vi "Exit if Runtime.vi"(3 "Top Level VI reference":refnum<vi>) -> ()   [LabVIEW 2026]
panel:
  in  "error in (no error)":errorcluster
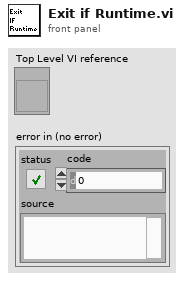
[diagram p1: front panel]
types:
  T1 = enum32{"invalid app kind", "Development System", "Run Time System", "Student Edition", "Embedded LabVIEW", "Evaluation", "Custom"}
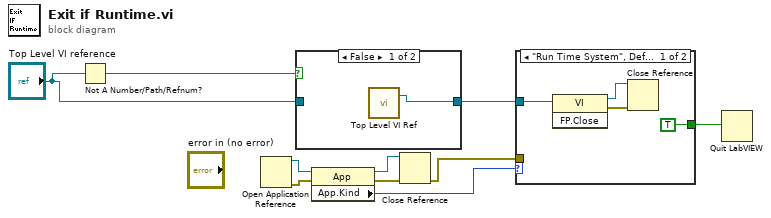
[diagram p0: block diagram]
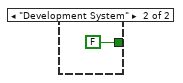
[diagram p2: hidden frame]
diagram:
  n1 = Not A Number/Path/Refnum?(number/path/refnum="Top Level VI reference") -> (NaN/Path/Refnum?=w10:bool)
  n2 = Open Application Reference() -> (0:w4:errorcluster, 3:w3:refnum<vi>)  [unwired: 4 in]
  n3 = case shown="False" w10 {
    tunnel: "Top Level VI reference" -> [_ w12]
    tunnel: [w11 w12] -> w2
    frame False {
      n4 = call "Top Level VI Ref.vi"() -> ("Top Level VI reference"=w11:refnum<vi>)  [unwired: 3 in]
    }
    frame True {
    }
  }
  n5 = property class="App"(reference=w3, error in=w4) -> (reference out=w5:refnum<vi>, error out=w8:errorcluster, "App.Kind"=w7:T1)
  n6 = Close Reference(reference=w5, error in (no error)=w8) -> (error out=w6:errorcluster)
  n7 = case shown="\"Run Time System\", Default" w7 {
    tunnel: w6 -> [_ _]
    tunnel: w2 -> [w16 _]
    tunnel: [TRUE FALSE] -> w1
    frame "Run Time System", Default {
      n8 = invoke class="VI" method="FP.Close"(reference=w16) -> (reference out=w14:refnum<vi>, error out=w15:errorcluster)  [unwired: 2 in, 1 out]
      n9 = Close Reference(reference=w14, error in (no error)=w15) -> ()  [unwired: 1 out]
    }
    frame "Development System" {
    }
  }
  n10 = Quit LabVIEW(quit? (T)=w1) -> ()
